vi "FGVTimer.vi"(8 "error in":errorcluster, 10 "set timer":dbl=-1.0, 11 "Reset":bool) -> (0 "error out":errorcluster, 2 "Elapsed?":bool, 3 "Time Elapsed":dbl)   [LabVIEW 2019]
doc: "Timer semplice che si basa su un numero random come limite di tempo massimo"
uses:
  <vilib>/numeric/Random Number (Range) DBL.vi
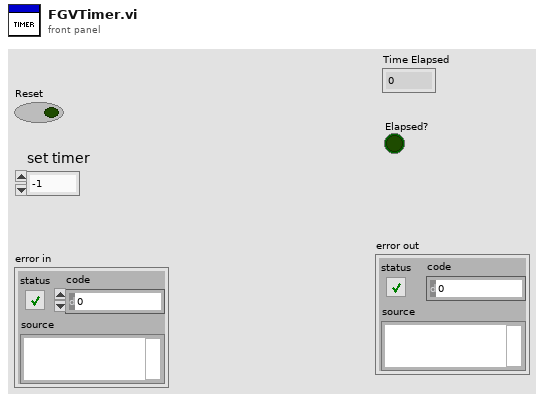
[diagram p1: front panel]
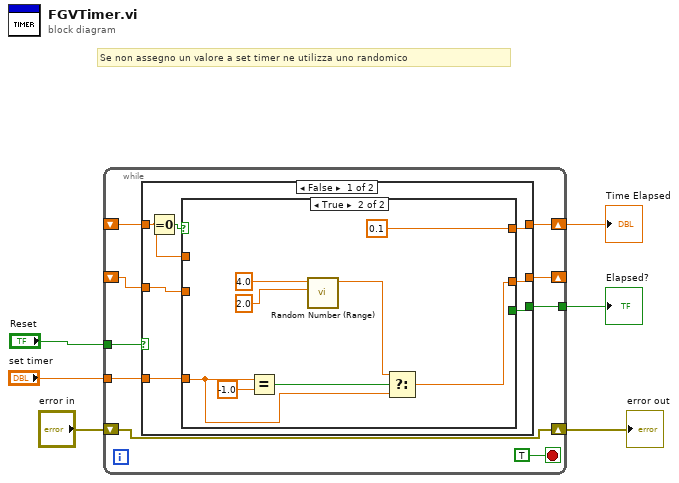
[diagram p0: block diagram]
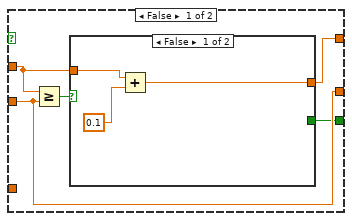
[diagram p2: hidden frame]
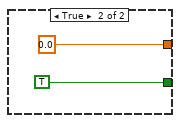
[diagram p3: hidden frame]
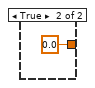
[diagram p4: hidden frame]
diagram:
  # "Se non assegno un valore a set timer ne utilizza uno randomico"
  n1 = while {
    shift-right: [w14] -> w6
    shift-left: _ -> [w13]
    shift-right: [w12] -> _
    shift-left: _ -> [w11]
    tunnel: [w10] -> w5
    shift-right: [w9] -> w3
    shift-left: "error in" -> [w9]
    tunnel: "Reset" -> [w8]
    tunnel: "set timer" -> [w7]
    stop <- TRUE stop-if-true
    n2 = case shown="False" w8 {
      tunnel: [w22 0.0] -> w14
      tunnel: w13 -> [w20 _]
      tunnel: [w19 _] -> w12
      tunnel: w11 -> [w18 _]
      tunnel: [w17 _] -> w10
      tunnel: w7 -> [w16 _]
      frame False {
        n3 = Equal To 0?(x=w20) -> (x = 0?=w21:bool)
        n4 = case shown="True" w21 {
          tunnel: [w25 0.1] -> w22
          tunnel: w20 -> [w26 _]
          tunnel: [w24 w35] -> w19
          tunnel: w18 -> [w24 _]
          tunnel: [w23 _] -> w17
          tunnel: w16 -> [_ w33]
          frame False {
            n5 = Greater Or Equal?(x=w26, y=w24) -> (x >= y?=w27:bool)
            n6 = case shown="False" w27 {
              tunnel: w26 -> [w30 _]
              tunnel: [w28 0.0] -> w25
              tunnel: [_ TRUE] -> w23
              frame False {
                n7 = Add(x=w30, y=0.1) -> (x+y=w28:dbl)
              }
              frame True {
              }
            }
          }
          frame True {
            n8 = Equal?(x=w33, y=-1.0) -> (x = y?=w36:bool)
            n9 = call-poly <vilib>:"Random Number (Range).vi"("lower bound (0)"=2.0, "upper bound (100)"=4.0) -> ("number"=w34:dbl)  [unwired: 9 in]
            n10 = Select(t=w34, s=w36, f=w33) -> (s? t:f=w35:dbl)
          }
        }
      }
      frame True {
      }
    }
  }
  "Time Elapsed" <- w6
  "Elapsed?" <- w5
  "error out" <- w3
